vi "outputPIP.vi"   [LabVIEW 2018]
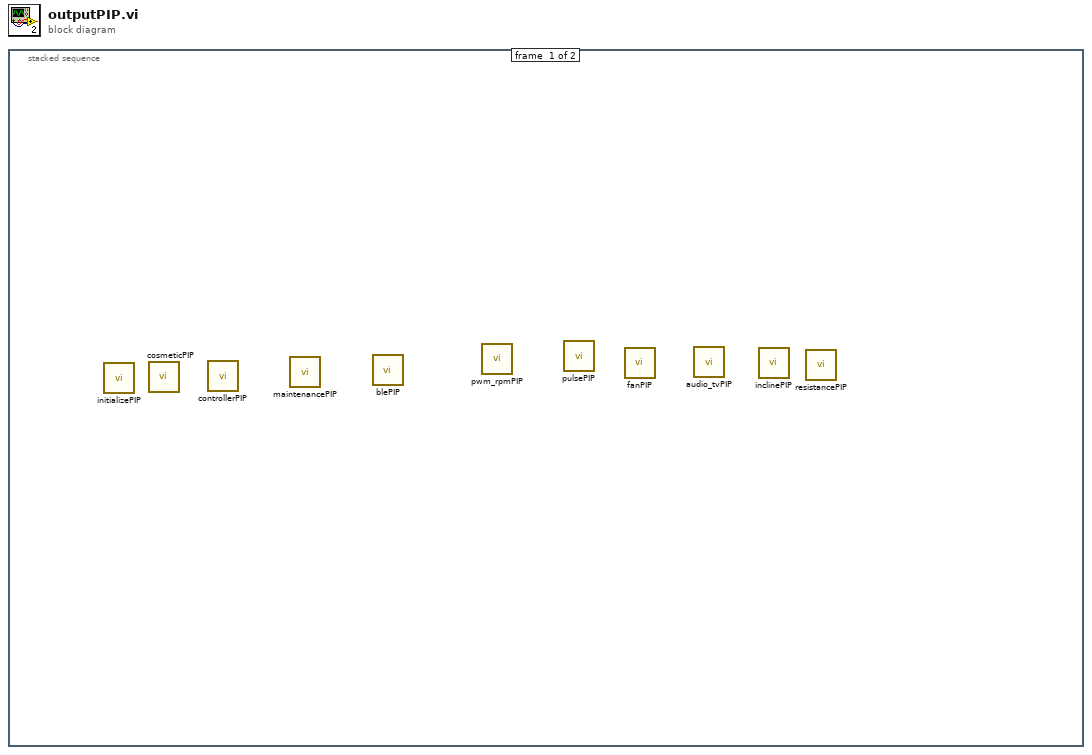
[diagram p0: block diagram]
diagram:
  n1 = stacked-sequence {
    frame #0 {
      n2 = call "initializePIP.vi"() -> ()  [unwired: 9 in, 3 out]
      n3 = call "cosmeticPIP.vi"() -> ()  [unwired: 10 in, 2 out]
      n4 = call "controllerPIP.vi"() -> ()  [unwired: 11 in, 5 out]
      n5 = call "maintenancePIP.vi"() -> ()  [unwired: 10 in, 2 out]
      n6 = call "blePIP.vi"() -> ()  [unwired: 12 in]
      n7 = call "pwm_rpmPIP.vi"() -> ()  [unwired: 10 in, 2 out]
      n8 = call "pulsePIP.vi"() -> ()  [unwired: 10 in, 2 out]
      n9 = call "fanPIP.vi"() -> ()  [unwired: 10 in, 2 out]
      n10 = call "audio_tvPIP.vi"() -> ()  [unwired: 9 in, 3 out]
      n11 = call "inclinePIP.vi"() -> ()  [unwired: 10 in, 2 out]
      n12 = call "resistancePIP.vi"() -> ()  [unwired: 10 in, 2 out]
    }
    frame #1 {
    }
  }
